vi "AppendPathSeparator.vi"(8 "Path separator (\\)":string="\\", 11 "Path":string) -> (0 "Dup path without separator":string, 3 "Dup path with separator":string)   [LabVIEW 2015]
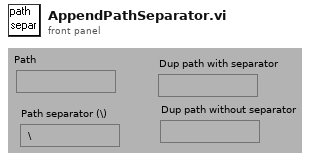
[diagram p1: front panel]
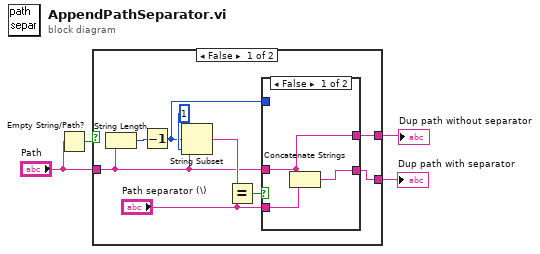
[diagram p0: block diagram]
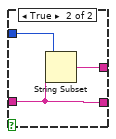
[diagram p2: hidden frame]
diagram:
  n1 = Empty String/Path?(string/path="Path") -> (empty?=w3:bool)
  n2 = case shown="False" w3 {
    tunnel: "Path" -> [w9 w20]
    tunnel: [w7 w20] -> w2
    tunnel: [w5 w20] -> w1
    frame False {
      n3 = String Length(string=w9) -> (length=w13:i32)
      n4 = Decrement(x=w13) -> (x-1=w6:i32)
      n5 = String Subset(string=w9, offset (0)=w6, length (rest)=1 ("length")) -> (substring=w11:string)
      n6 = Equal?(x=w11, y="Path separator (\\)") -> (x = y?=w10:bool)
      n7 = case shown="False" w10 {
        tunnel: w9 -> [w14 w18]
        tunnel: "Path separator (\\)" -> [w16 _]
        tunnel: [w15 w18] -> w7
        tunnel: w6 -> [_ w19]
        tunnel: [w14 w17] -> w5
        frame False {
          n8 = Concatenate Strings(w14, w16) -> (w15:string)
        }
        frame True {
          n9 = String Subset(string=w18, length (rest)=w19) -> (substring=w17:string)  [unwired: 1 out]
        }
      }
    }
    frame True {
    }
  }
  "Dup path with separator" <- w2
  "Dup path without separator" <- w1
